vi "array_shit.vi"() -> ()   [LabVIEW 2013]
panel:
  out "output array":i32[](array[numeric])
  out "array":i32[][](array[numeric])
  out "subarray":i32[][](array[numeric])
  in  "Reihe":i32
  in  "length 2":i32
  in  "length":i32
  in  "Spalte":i32
  out "String":string
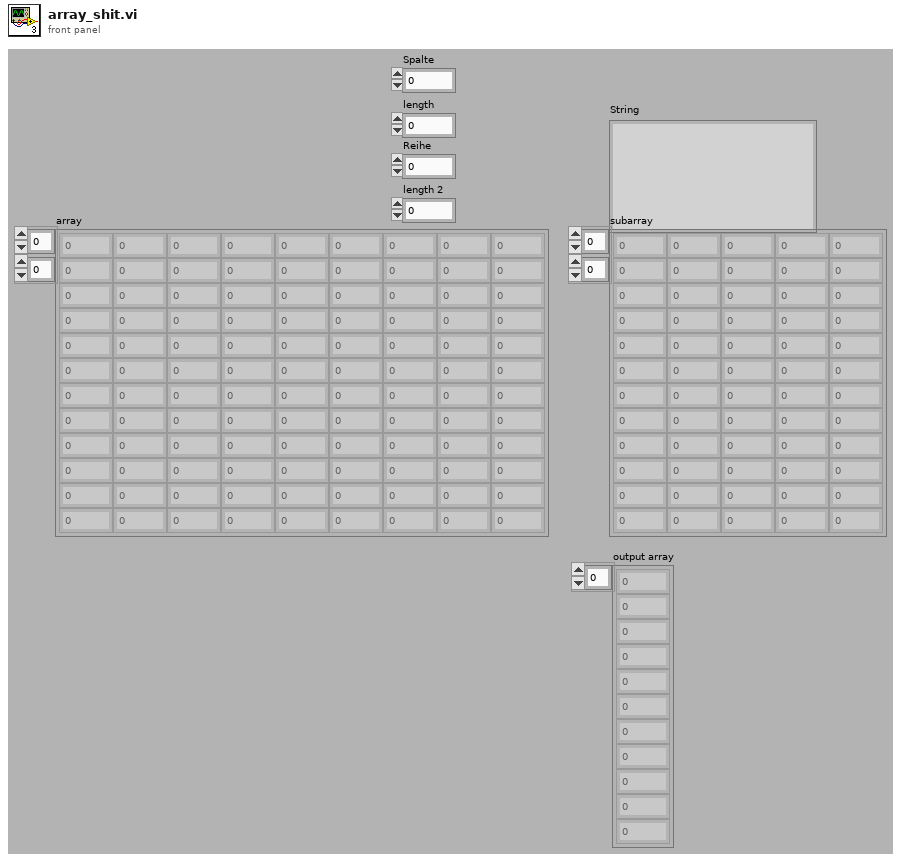
[diagram p1: front panel]
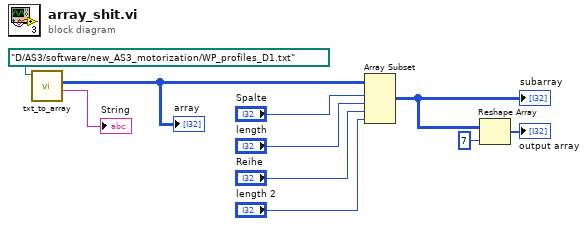
[diagram p0: block diagram]
diagram:
  n1 = call "txt_to_array.vi"("file (use dialog)"=path "D:/AS3/software/new_AS3_motorization/WP_profiles_D1.txt") -> ("String"=→"String":string, "array"=w9:i32[][])  [unwired: 8 in, 1 out]
  "array" <- w9
  n2 = Array Subset(array=w9, index (row)="Spalte", length (row)="length", index (col)="Reihe", length (col)="length 2") -> (w3:i32[][])
  "subarray" <- w3
  n3 = Reshape Array(w3, 7 ("dimension size")) -> (→"output array":i32[])
